vi "FRCts20_WebMethods_Convert_SingleEvent.vi"(8 "error in (no error)":errorcluster, 10 "ClosedRequestsData":T1, 11 "Event Out":T2) -> (0 "error out":errorcluster, 3 "Event":T4)   [LabVIEW 2014, in "FRCts20_WebMethods.lvlib"]
uses:
  FRCts20_WebMethods.lvlib
  ESP Engine/source/VI Source/TypeDefs/FRCts20_EspEngine_Event.ctl
  Web Method Public Interface/FRCts20_WebMethods_ctl_singleEvent.ctl
  Web Method Public Interface/FRCts20_WebMethods_ctl_teamIdentifier.ctl
  Backend/source/VI Source/FRCts20_Backend_API/FRCts20_Backend_API_Event.ctl
  Backend/source/VI Source/FRCts20_Backend_API/FRCts20_Backend_API_SW.ctl
  Backend/source/VI Source/FRCts20_Backend_API/FRCts20_Backend_API_ClosedRequests.ctl
  ESP Engine/source/VI Source/FRCts20_EspEngine.lvlib
  Backend/source/VI Source/FRCts20_Backend_API/FRCts20_Backend_API.lvlib
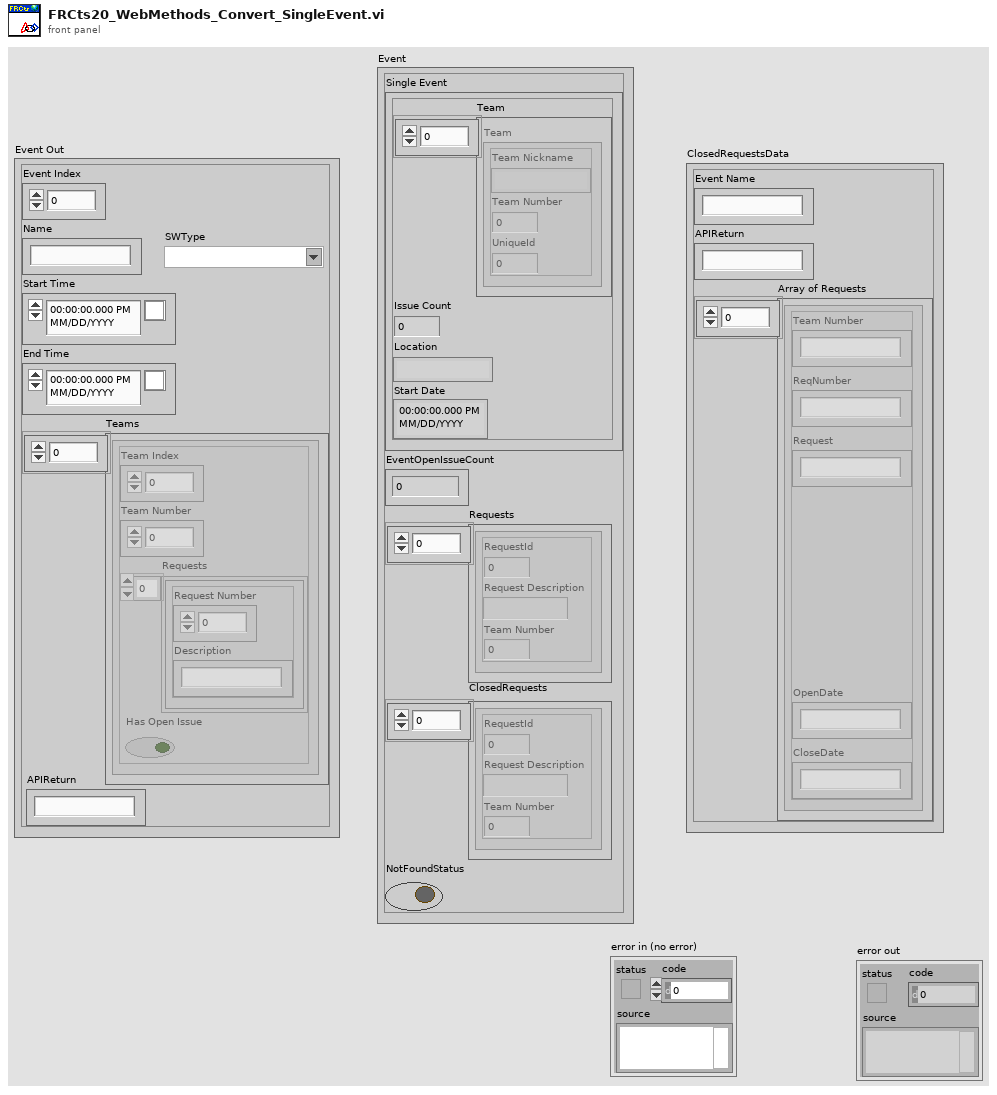
[diagram p1: front panel]
types:
  T1 = typedef "FRCts20_Backend_API_ClosedRequests.ctl" = cluster{"Event Name":string, "APIReturn":string, "Array of Requests":cluster{"Team Number":string, "ReqNumber":string, "Request":string, "OpenDate":string, "CloseDate":string}[]}
  T2 = typedef "FRCts20_Backend_Engine.lvlib/FRCts20_Backend_API.lvlib/FRCts20_Backend_API_Event.ctl" = cluster{"Event Index":u32, "Name":string, "Start Time":timestamp, "End Time":timestamp, "Teams":cluster{"Team Index":u32, "Team Number":u32, "Requests":cluster{"Request Number":u32, "Description":string}[], "Has Open Issue":bool}[], "SWType":T3, "APIReturn":string}
  T3 = typedef "FRCts20_Backend_Engine.lvlib/FRCts20_Backend_API.lvlib/FRCts20_Backend_API_SW.ctl" = string
  T4 = typedef "FRCts20_EspEngine.lvlib/FRCts20_EspEngine_Event.ctl" = cluster{"Single Event":T5, "EventOpenIssueCount":i16, "Requests":cluster{"RequestId":i32, "Request Description":string, "Team Number":i32}[], "ClosedRequests":cluster{"RequestId":i32, "Request Description":string, "Team Number":i32}[], "NotFoundStatus":bool}
  T5 = typedef "FRCts20_WebMethods.lvlib/FRCts20_WebMethods_ctl_singleEvent.ctl" = cluster{"Team":T6[], "Issue Count":i32, "Location":string, "Start Date ":timestamp}
  T6 = typedef "FRCts20_WebMethods.lvlib/FRCts20_WebMethods_ctl_teamIdentifier.ctl" = cluster{"Team Nickname":string, "Team Number ":u32, "UniqueId":u32}
  T7 = cluster{"RequestId":i32, "Request Description":string, "Team Number":i32}
  T8 = cluster{"Team Number":string, "ReqNumber":string, "Request":string, "OpenDate":string, "CloseDate":string}[]
  T9 = cluster{"Team Index":u32, "Team Number":u32, "Requests":cluster{"Request Number":u32, "Description":string}[], "Has Open Issue":bool}[]
  T10 = cluster{"Request Number":u32, "Description":string}[]
  T11 = cluster{"RequestId":i32, "Request Description":string, "Team Number":i32}[]
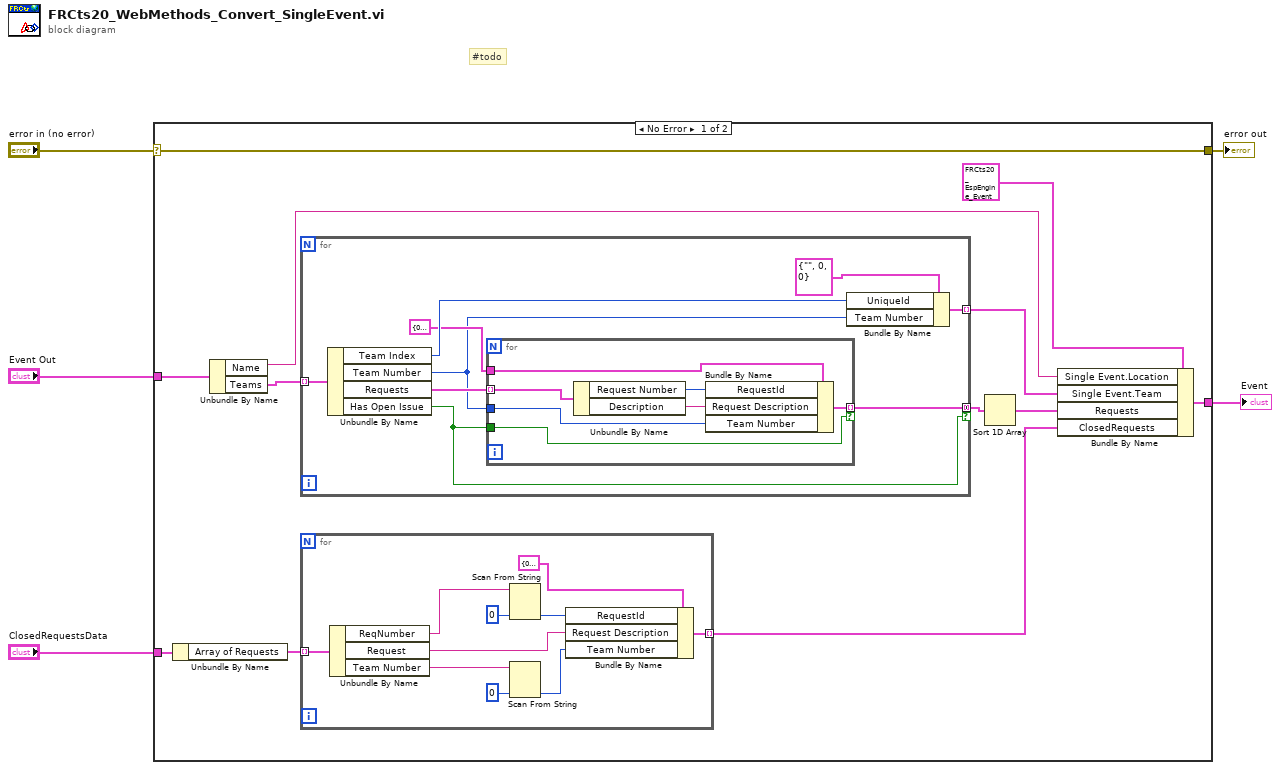
[diagram p0: block diagram]
diagram:
  # "#todo"
  n1 = case shown="No Error" "error in (no error)" {
    selector: "error in (no error)" -> [w10 w44]
    tunnel: [w10 w44] -> w5
    tunnel: "Event Out" -> [w12 _]
    tunnel: [w11 _] -> w2
    tunnel: "ClosedRequestsData" -> [w9 _]
    frame No Error {
      n2 = Unbundle By Name(w9) -> ("Array of Requests"=w8:T8)
      n3 = Unbundle By Name(w12) -> ("Name"=w16:string, "Teams"=w15:T9)
      n4 = for {
        tunnel: w15 -> [w36] mode=indexing
        tunnel: [w33] -> w14 mode=indexing
        tunnel: [w28] -> w13 mode=concatenating if=w29
        n5 = Unbundle By Name(w36) -> ("Team Index"=w34:u32, "Team Number"=w30:u32, "Requests"=w31:T10, "Has Open Issue"=w29:bool)
        n6 = for {
          tunnel: T7 {"RequestId"=0, "Request Description"="", "Team Number"=0} ("Request") -> [w43]
          tunnel: [w42] -> w28 mode=indexing if=w37
          tunnel: w31 -> [w41] mode=indexing
          tunnel: w30 -> [w38]
          tunnel: w29 -> [w37]
          n7 = Unbundle By Name(w41) -> ("Request Number"=w40:u32, "Description"=w39:string)
          n8 = Bundle By Name(cluster=w43, "RequestId"=w40, "Request Description"=w39, "Team Number"=w38) -> (w42:T7)
        }
        n9 = Bundle By Name(cluster=T6 {"Team Nickname"="", "Team Number "=0, "UniqueId"=0} ("Team"), "UniqueId"=w34, "Team Number"=w30) -> (w33:T6)
      }
      n10 = for {
        tunnel: w8 -> [w26] mode=indexing
        tunnel: [w18] -> w7 mode=indexing
        n11 = Unbundle By Name(w26) -> ("ReqNumber"=w25:string, "Request"=w22:string, "Team Number"=w20:string)
        n12 = Scan From String(input string=w25, default 1=0 ("RequestId")) -> (output 1=w23:i32)  [unwired: 3 in, 3 out]
        n13 = Scan From String(input string=w20, default 1=0 ("RequestId")) -> (output 1=w19:i32)  [unwired: 3 in, 3 out]
        n14 = Bundle By Name(cluster=T7 {"RequestId"=0, "Request Description"="", "Team Number"=0} ("Request"), "RequestId"=w23, "Request Description"=w22, "Team Number"=w19) -> (w18:T7)
      }
      n15 = Sort 1D Array(array=w13) -> (sorted array=w6:T11)
      n16 = Bundle By Name(cluster=T4 {"Single Event"={"Team"=[], "Issue Count"=0, "Location"="", "Start Date "=timestamp(0 s since 1904-01-01)}, "EventOpenIssueCount"=0, "Requests"=[], "ClosedRequests"=[], "NotFoundStatus"=FALSE} ("Event"), "Single Event.Location"=w16, "Single Event.Team"=w14, "Requests"=w6, "ClosedRequests"=w7) -> (w11:T4)
    }
    frame Error {
    }
  }
  "Event" <- w2
  "error out" <- w5
